vi "PhotonPoseEstimator_SetReferencePose_Pose2d.vi"(9 "ReferencePose2D":T2={"TRANSLATION"={"X"=0.0, "Y"=0.0}, "ROTATION"={"VALUE"=0.0, "COS"=1.0, "SIN"=0.0}} {"ROTATION"."SIN" format="%13.4f"; "ROTATION"."COS" format="%13.4f"; "ROTATION"."VALUE" format="%13.4f"; "TRANSLATION"."Y" format="%14.3f"; "TRANSLATION"."X" format="%14.3f"}, 11 "PhotonPoseEstimator":T1) -> (3 "out PhotonPoseEstimator":T1)   [LabVIEW 2019, in "PhotonVisionLib.lvlib"]
doc: "Set the reference pose from the PhotonPoseEstimator cluster.\n\nInputs: \n -- PhotonVisionPoseEstimator -- cluster -- The estimator.\n -- referencePose -- Pose2d -- This is the reference pose being used by the Photon Pose Estimator. Often this would be set the the current Pose calculated by the robot's odometry.\n\nOutputs:\n -- PhotonVisionPoseEstimator -- cluster -- The updated estimator."
uses:
  PhotonVisionLib.lvlib
  TypeDef/PhotonPoseEstimatorType.ctl
  <vilib>/Rock Robotics/WPI/ThirdParty/JAS_Junk/TrajLib/TypeDef/POSE3D.ctl
  <vilib>/Rock Robotics/WPI/ThirdParty/JAS_Junk/TrajLib/TypeDef/TRANSLATION3D.ctl
  <vilib>/Rock Robotics/WPI/ThirdParty/JAS_Junk/TrajLib/TypeDef/ROTATION3D.ctl
  <vilib>/Rock Robotics/WPI/ThirdParty/JAS_Junk/TrajLib/TypeDef/QUATERNION.ctl
  <vilib>/Rock Robotics/WPI/ThirdParty/JAS_Junk/TrajLib/TypeDef/AprilTagFieldLayout.ctl
  <vilib>/Rock Robotics/WPI/ThirdParty/JAS_Junk/TrajLib/TypeDef/AprilTag.ctl
  <vilib>/Rock Robotics/WPI/ThirdParty/JAS_Junk/TrajLib/Enum/AprilTagFieldLayoutOrignPosition_ENUM.ctl
  Enum/PhotonPoseStrategy_ENUM.ctl
  <vilib>/Rock Robotics/WPI/ThirdParty/JAS_Junk/TrajLib/TypeDef/TRANSFORM3D.ctl
  TypeDef/PhotonTargetModel.ctl
  <vilib>/Rock Robotics/WPI/ThirdParty/JAS_Junk/TrajLib/TypeDef/POSE2D.ctl
  <vilib>/Rock Robotics/WPI/ThirdParty/JAS_Junk/TrajLib/TypeDef/TRANSLATION2D.ctl
  <vilib>/Rock Robotics/WPI/ThirdParty/JAS_Junk/TrajLib/TypeDef/ROTATION2D.ctl
  <vilib>/Rock Robotics/WPI/ThirdParty/JAS_Junk/TrajLib/VI/Pose3d_New_Trans3dRot3d.vi
  <vilib>/Rock Robotics/WPI/ThirdParty/JAS_Junk/TrajLib/VI/Translation3d_Create.vi
  <vilib>/Rock Robotics/WPI/ThirdParty/JAS_Junk/TrajLib/VI/Rotation3d_Create_RollPitchYaw.vi
  <vilib>/Rock Robotics/WPI/ThirdParty/JAS_Junk/TrajLib/Pose2d_getXYAngle.vi
  <vilib>/Rock Robotics/WPI/ThirdParty/JAS_Junk/TrajLib/VI/Quaternion_New.vi
  <vilib>/Rock Robotics/WPI/ThirdParty/JAS_Junk/TrajLib/Trajectory_Library.lvlib
  Ref/PhotonPoseEstimator_REF.ctl
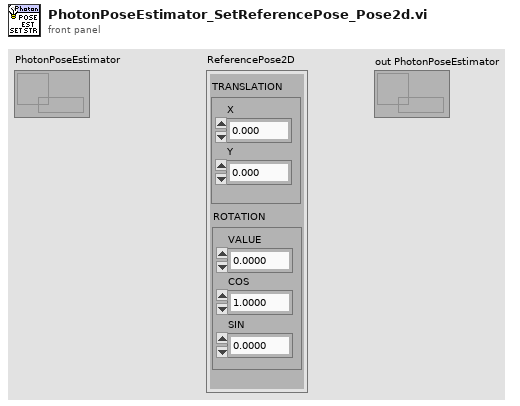
[diagram p1: front panel]
types:
  T1 = typedef "PhotonVisionLib.lvlib/PhotonPoseEstimator_REF.ctl" = refnum<data-value>
  T2 = typedef "Trajectory_Library.lvlib/POSE2D.ctl" = cluster{"TRANSLATION":T3, "ROTATION":T4}
  T3 = typedef "Trajectory_Library.lvlib/TRANSLATION2D.ctl" = cluster{"X":dbl, "Y":dbl}
  T4 = typedef "Trajectory_Library.lvlib/ROTATION2D.ctl" = cluster{"VALUE":dbl, "COS":dbl, "SIN":dbl}
  T5 = typedef "PhotonVisionLib.lvlib/PhotonPoseEstimatorType.ctl" = cluster{"LastPose":T6, "ReferencePose":T6, "FieldTags":T10, "PrimaryStratety":T13, "Camera":string, "RobotToCamera":T14, "ReportedErrors":dbl[], "HighestAmbiguity":dbl, "MultiTagFallbackStrategy":T13, "PoseCacheTimeoutSec":dbl, "PhotonTargetModel":T15, "BaseNTName":string}
  T6 = typedef "Trajectory_Library.lvlib/POSE3D.ctl" = cluster{"Translation3d":T7, "Rotation3d":T8}
  T7 = typedef "Trajectory_Library.lvlib/TRANSLATION3D.ctl" = cluster{"X":dbl, "Y":dbl, "Z":dbl}
  T8 = typedef "Trajectory_Library.lvlib/ROTATION3D.ctl" = cluster{"Q_quaternion":T9}
  T9 = typedef "Trajectory_Library.lvlib/QUATERNION.ctl" = cluster{"R":dbl, "V":dbl[]}
  T10 = typedef "Trajectory_Library.lvlib/AprilTagFieldLayout.ctl" = cluster{"AprilTagMap":map{i32, T11}, "FieldLength":dbl, "FieldWidth":dbl, "OriginPosition ":T12, "OriginPose3d":T6}
  T11 = typedef "Trajectory_Library.lvlib/AprilTag.ctl" = cluster{"ID":i32, "POSE3D":T6}
  T12 = typedef "Trajectory_Library.lvlib/AprilTagFieldLayoutOrignPosition_ENUM.ctl" = enum16{"kBlueAllianceWallRightSide,", "kRedAllianceWallRightSide,"}
  T13 = typedef "PhotonVisionLib.lvlib/PhotonPoseStrategy_ENUM.ctl" = enum16{"LOWEST_AMBIGUITY", "CLOSEST_TO_CAMERA_HEIGHT", "CLOSEST_TO_REFERENCE_POSE", "CLOSEST_TO_LAST_POSE", "AVERAGE_BEST_TARGETS", "MULTI_TAG_PNP_ON_COPROCESSOR", "MULTI_TAG_PNP_ON_RIO"}
  T14 = typedef "Trajectory_Library.lvlib/TRANSFORM3D.ctl" = cluster{"TRANSLATION3D":T7, "ROTATION3D":T8, "XF":bool}
  T15 = typedef "PhotonVisionLib.lvlib/PhotonTargetModel.ctl" = cluster{"Vertices":T7[], "IsPlaner":bool, "IsSpherical":bool}
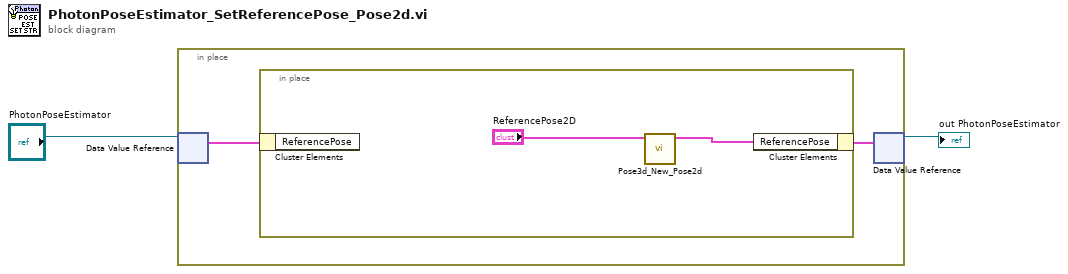
[diagram p0: block diagram]
diagram:
  n1 = in-place {
    n2 = in-place-dvr #1("PhotonPoseEstimator") -> (w4:T5)  [unwired: 1 out]
    n3 = in-place {
      n4 = in-place-cluster #2(w4) -> ()  [unwired: 1 out]
      n5 = call <vilib>:"Pose3d_New_Pose2d.vi"("in POSE2D"="ReferencePose2D") -> ("out Pose3d"=w5:T6)  [unwired: 10 in]
      n6 = in-place-cluster #2("ReferencePose"=w5) -> (w3:T5)
    }
    n7 = in-place-dvr #1(w3) -> (→"out PhotonPoseEstimator":T1)  [unwired: 1 out]
  }
